vi "Save_Info.vi"(8 "error in (no error)":errorcluster, 11 "AB_Build in":refnum<class "AB_Build.lvclass">) -> (0 "error out":errorcluster, 3 "AB_Build out":refnum<class "AB_Build.lvclass">)   [LabVIEW 2020, in "AB_Build.lvclass"]
uses:
  <vilib>/AppBuilder/AB_Classes/Build/AB_Build.lvclass
  <vilib>/AppBuilder/AB_Classes/Build/AB_Build.lvclass/AB_Build.ctl
  <vilib>/AppBuilder/RW_Project/AB_RW_Project_Build_Data.ctl
  <vilib>/AppBuilder/RW_Project/AB_RW_Project_PropBag_Action.ctl
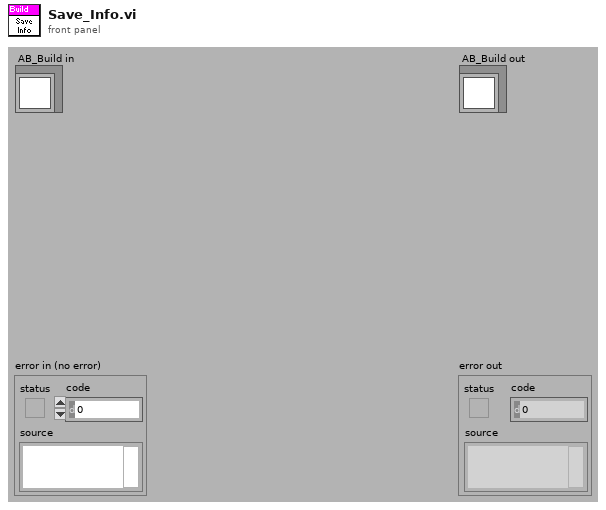
[diagram p1: front panel]
types:
  T1 = typedef "AB_RW_Project_PropBag_Action.ctl" = enum16{"read", "write", "clear", "readPrevious", "writePrevious", "clearPrevious"}
  T2 = typedef "AB_RW_Project_Build_Data.ctl" = cluster{"buildSpecName":string, "buildSpecDescription":string, "excludeTypedefs":bool, "excludePolymorphicVIs":bool, "excludeLibraryItems":bool, "modifyLibraryFile":bool, "defaultLanguage":string, "supportedLanguages":string[], "excludedDirectories":path[], "userLog_Path":path, "preActionVIID":string, "postActionVIID":string, "localDest_Path":path, "targetDest_Path":path, "removeVIObject":u16, "previewCache_ID":string, "buildCache_ID":string, "excludeInlineSubVIs":bool, "bldVersion":cluster{"major":u16, "minor":u16, "patch":u16, "build":u16}, "autoIncrement":bool, "excludeDependentPPLs":bool, "excludeDependentDLLs":bool}
  T3 = typedef "ItemRef.ctl" = u64
  T4 = cluster{"major":u16, "minor":u16, "patch":u16, "build":u16}
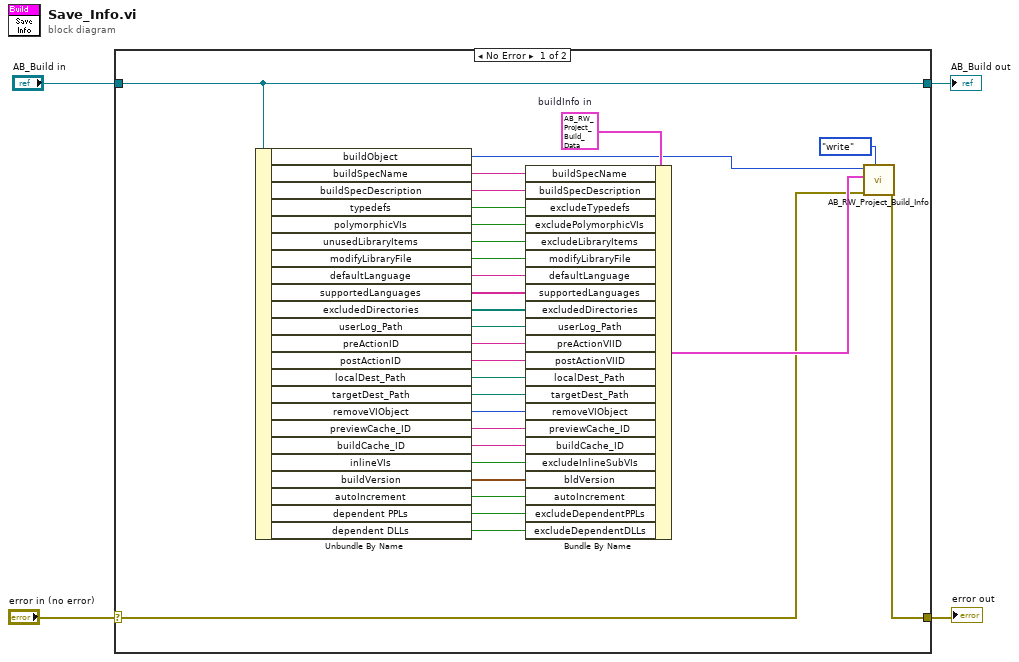
[diagram p0: block diagram]
diagram:
  n1 = case shown="No Error" "error in (no error)" {
    selector: "error in (no error)" -> [w10 w35]
    tunnel: [w32 w35] -> w3
    tunnel: [w24 w34] -> w1
    tunnel: "AB_Build in" -> [w24 w34]
    frame No Error {
      w31 = T2 {"buildSpecName"="", "buildSpecDescription"="", "excludeTypedefs"=FALSE, "excludePolymorphicVIs"=FALSE, "excludeLibraryItems"=FALSE, "modifyLibraryFile"=FALSE, "defaultLanguage"="", "supportedLanguages"=[], "excludedDirectories"=[], "userLog_Path"=path "", "preActionVIID"="", "postActionVIID"="", "localDest_Path"=path "", "targetDest_Path"=path "", "removeVIObject"=0, "previewCache_ID"="", "buildCache_ID"="", "excludeInlineSubVIs"=FALSE, "bldVersion"={"major"=0, "minor"=0, "patch"=0, "build"=0}, "autoIncrement"=FALSE, "excludeDependentPPLs"=FALSE, "excludeDependentDLLs"=FALSE}  # buildInfo in
      n2 = Unbundle By Name(w24) -> ("buildObject"=w9:T3, "buildSpecName"=w30:string, "buildSpecDescription"=w20:string, "typedefs"=w29:bool, "polymorphicVIs"=w23:bool, "unusedLibraryItems"=w22:bool, "modifyLibraryFile"=w21:bool, "defaultLanguage"=w28:string, "supportedLanguages"=w27:string[], "excludedDirectories"=w26:path[], "userLog_Path"=w19:path, "preActionID"=w18:string, "postActionID"=w17:string, "localDest_Path"=w16:path, "targetDest_Path"=w15:path, "removeVIObject"=w14:u16, "previewCache_ID"=w13:string, "buildCache_ID"=w12:string, "inlineVIs"=w11:bool, "buildVersion"=w8:T4, "autoIncrement"=w7:bool, "dependent PPLs"=w6:bool, "dependent DLLs"=w5:bool)
      n3 = Bundle By Name(cluster=w31, "buildSpecName"=w30, "buildSpecDescription"=w20, "excludeTypedefs"=w29, "excludePolymorphicVIs"=w23, "excludeLibraryItems"=w22, "modifyLibraryFile"=w21, "defaultLanguage"=w28, "supportedLanguages"=w27, "excludedDirectories"=w26, "userLog_Path"=w19, "preActionVIID"=w18, "postActionVIID"=w17, "localDest_Path"=w16, "targetDest_Path"=w15, "removeVIObject"=w14, "previewCache_ID"=w13, "buildCache_ID"=w12, "excludeInlineSubVIs"=w11, "bldVersion"=w8, "autoIncrement"=w7, "excludeDependentPPLs"=w6, "excludeDependentDLLs"=w5) -> (w25:T2)
      n4 = call <vilib>:"AB_RW_Project_Build_Info.vi"("action"=AB_RW_Project_PropBag_Action."write", "error in (no error)"=w10, "buildInfo in"=w25, "Object In"=w9) -> ("error out"=w32:errorcluster)  [unwired: 7 out]
    }
    frame Error {
    }
  }
  "error out" <- w3
  "AB_Build out" <- w1
